vi "FeederTrend.vi"() -> ()   [LabVIEW 2025]
uses:
  <vilib>/Rock Robotics/Network Tables/NT Read Number.vi
  DashBoardGlobals.vi
panel:
  out "Feeder Speed Chart":T1(graph)
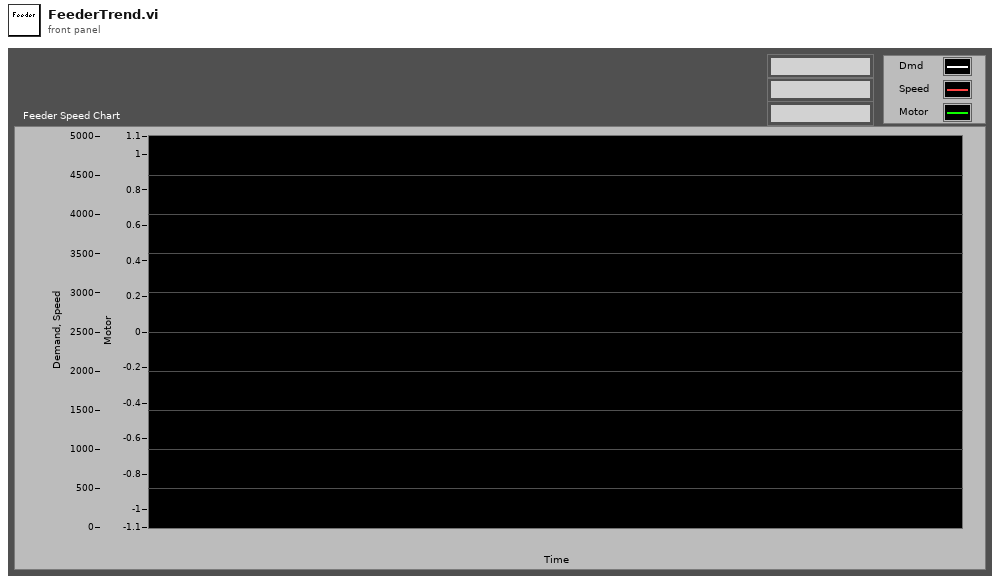
[diagram p1: front panel]
types:
  T1 = cluster{"TravSpdDmdFPS":dbl, "TravSpeedFPS":dbl, "TravMotDmd":dbl}
  T2 = enum8{"Tele-Op Disabled", "Tele-Op Enabled", "Auto Disabled", "Auto Enabled", "Test Disabled", "Test Enabled", "Disconnected", "No Code", "E-Stop"}
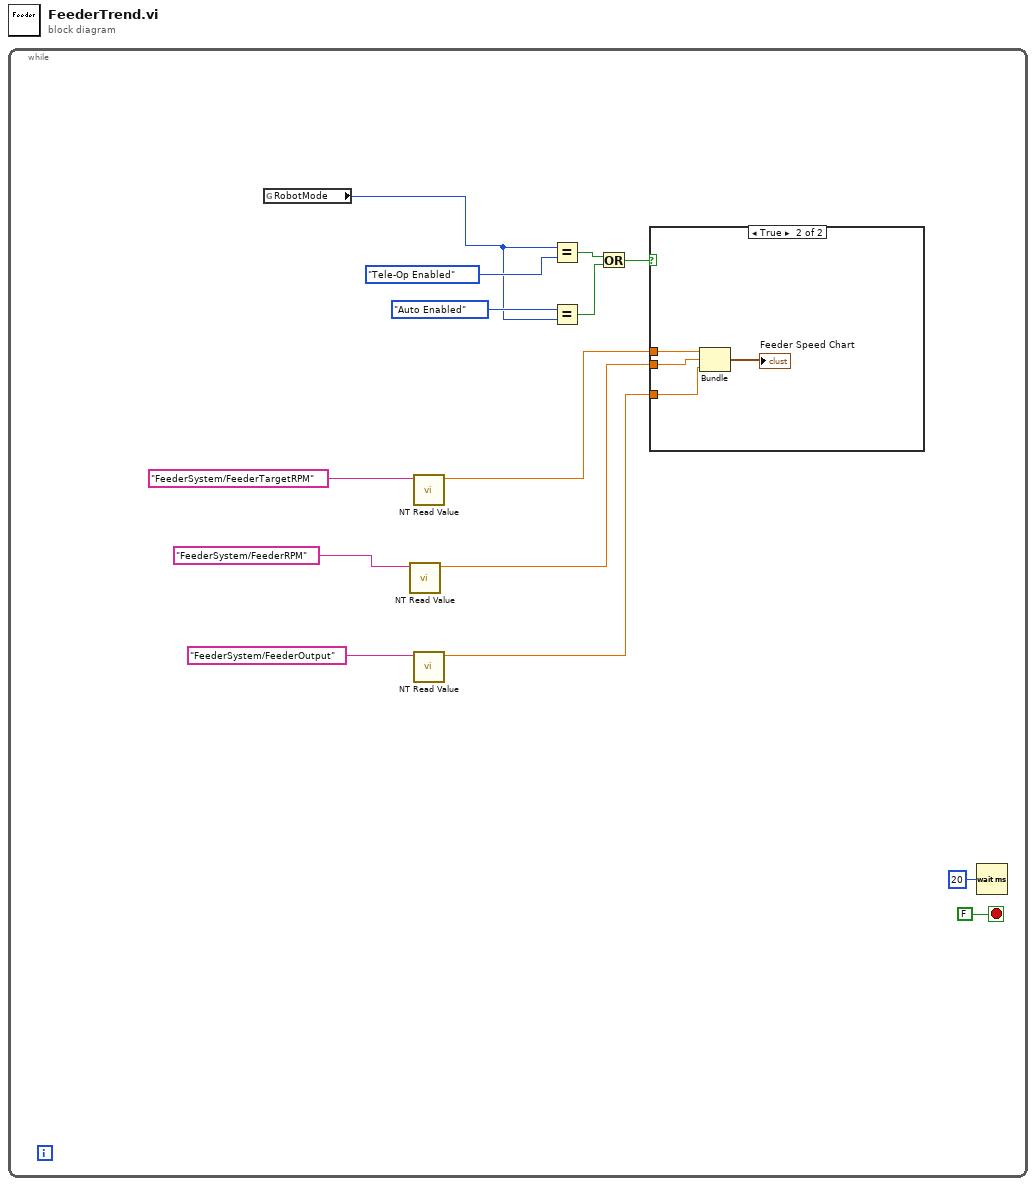
[diagram p0: block diagram]
diagram:
  n1 = while {
    stop <- FALSE stop-if-true
    n2 = global read "DashBoardGlobals.vi" "RobotMode"() -> (w7:T2)
    n3 = call-poly <vilib>:"NT Read Value.vi"("name"="FeederSystem/FeederRPM") -> ("value"=w2:dbl)  [unwired: 8 in, 2 out]
    n4 = call-poly <vilib>:"NT Read Value.vi"("name"="FeederSystem/FeederTargetRPM") -> ("value"=w3:dbl)  [unwired: 8 in, 2 out]
    n5 = call-poly <vilib>:"NT Read Value.vi"("name"="FeederSystem/FeederOutput") -> ("value"=w1:dbl)  [unwired: 8 in, 2 out]
    n6 = Equal?(x=w7, y=T2."Tele-Op Enabled") -> (x = y?=w10:bool)
    n7 = Equal?(x=T2."Auto Enabled" ("y"), y=w7) -> (x = y?=w9:bool)
    n8 = Or(x=w10, y=w9) -> (x .or. y?=w8:bool)
    n9 = case shown="True" w8 {
      tunnel: w3 -> [_ w18]
      tunnel: w2 -> [_ w17]
      tunnel: w1 -> [_ w16]
      frame False {
      }
      frame True {
        n10 = Bundle("value"=w18, "value"=w17, "value"=w16) -> (→"Feeder Speed Chart":cluster{"value":dbl, "value":dbl, "value":dbl})  [unwired: 1 in]
      }
    }
    n11 = Wait (ms)(milliseconds to wait=u32 20) -> ()  [unwired: 1 out]
  }
